vi "K2400_Initialize.vi"(1 "error in":errorcluster, 2 "RCL #":dbl format="%#_3g", 3 "Setup":bool=TRUE, 4 "address (24)":string="24") -> (0 "error out":errorcluster)   [LabVIEW 2021]
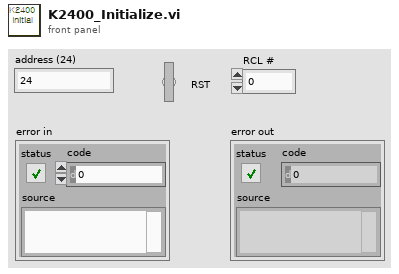
[diagram p1: front panel]
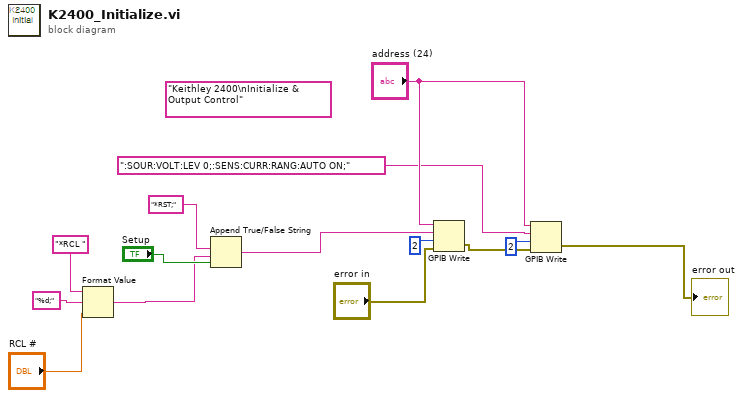
[diagram p0: block diagram]
diagram:
  (unwired) "Keithley 2400\nInitialize & Output Control"
  n1 = Format Value(string ("")="*RCL ", format string="%d;", value (0)="RCL #") -> (output string=w1:string)
  n2 = Append True/False String(1:"Setup", 2:w1, 3:"*RST;") -> (0:w3:string)  [unwired: 1 in]
  n3 = GPIB Write(0:"address (24)", 1:w3, 2:2, 3:"error in") -> (6:w7:errorcluster)  [unwired: 1 in, 1 out]
  n4 = GPIB Write(0:"address (24)", 1:":SOUR:VOLT:LEV 0;:SENS:CURR:RANG:AUTO ON;", 2:2, 3:w7) -> (6:→"error out":errorcluster)  [unwired: 1 in, 1 out]
